vi "calculate_angleXZ_and_angleYZ.vi"(2 "period [s]":dbl format="%#_13g", 3 "Previous angle (XZ, YZ)":dbl[](array[numeric]), 4 "Averaged rotation (XZ, YZ)":dbl[](array[numeric])) -> (0 "angleYZ":dbl, 1 "angleXZ":dbl)   [LabVIEW 2015]
doc: "Calcultes the current angle in XZ and YZ plane returning the value expressed in radians."
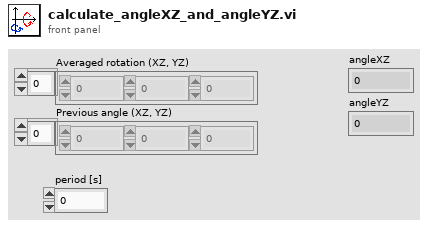
[diagram p1: front panel]
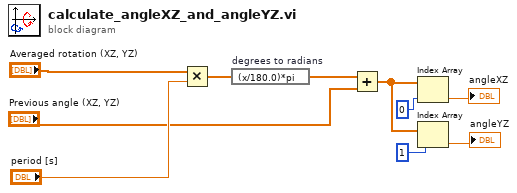
[diagram p0: block diagram]
diagram:
  n1 = Multiply(x="Averaged rotation (XZ, YZ)", y="period [s]") -> (x*y=w9:dbl[])
  n2 = expression code="(x/180.0)*pi" "degrees to radians"(w9) -> (w2:dbl[])
  n3 = Add(x=w2, y="Previous angle (XZ, YZ)") -> (x+y=w1:dbl[])
  n4 = Index Array(array=w1, index=0) -> (element=→"angleXZ":dbl)
  n5 = Index Array(array=w1, index=1) -> (element=→"angleYZ":dbl)
